vi "Create Queue.vi"() -> ()   [LabVIEW 2015]
uses:
  Core/HTTP Request/Region.ctl
  Core/HTTP Request/AWS Credentials.ctl
  Queue/Queue.lvclass
  Core/HTTP Request/HTTP Request.lvclass
panel:
  in  "Region":T1
  in  "Secret Key":string
  in  "Access Key":string
  in  "Queue Name":string
  # "Overview: Demonstrates how to create a new Amazon SQS queue.\nRequirements: LabVIEW AWS Toolkit and a registered Amazon AWS account\nInstructions:\n1. Specify the Access Key and Secret Key for your AWS account. You can create an account at http://aws.amazon.com.\n2. Specify a Region and Queue Name for the queue you want to create. Note that the queue name must be globally unique.\n3. Run the VI. Verify in the Amazon SQS console that the specified queue was created."
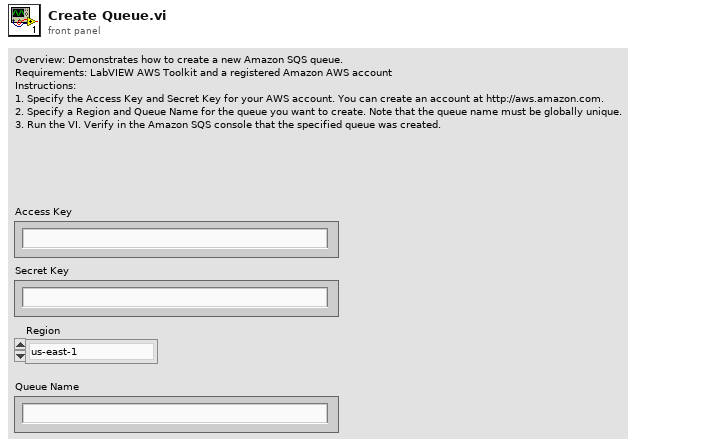
[diagram p1: front panel]
types:
  T1 = typedef "NI_AWS_Core.lvlib/HTTP Request.lvclass/Region.ctl" = enum16{"us-east-1", "us-east-2", "us-west-1", "us-west-2", "ap-northeast-1", "ap-northeast-2", "ap-southeast-1", "ap-southeast-2", "ca-central-1", "eu-central-1", "eu-west-1", "eu-west-2", "sa-east-1"}
  T2 = typedef "NI_AWS_Core.lvlib/HTTP Request.lvclass/AWS Credentials.ctl" = cluster{"Access Key":string, "Secret Key":string}
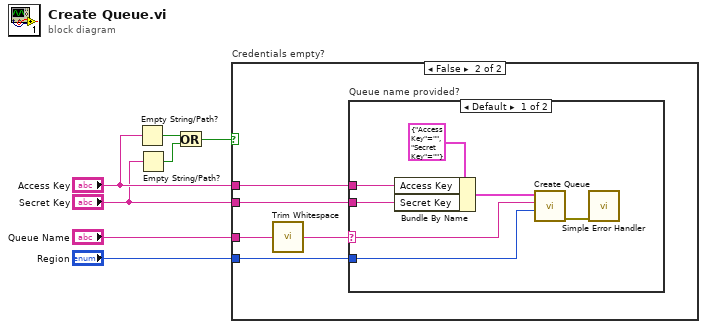
[diagram p0: block diagram]
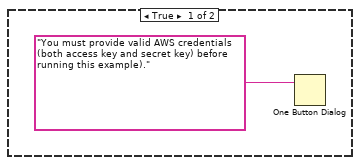
[diagram p2: hidden frame]
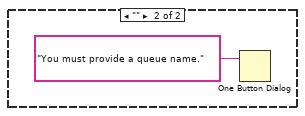
[diagram p3: hidden frame]
diagram:
  n1 = Empty String/Path?(string/path="Access Key") -> (empty?=w7:bool)
  n2 = Empty String/Path?(string/path="Secret Key") -> (empty?=w6:bool)
  n3 = Or(x=w7, y=w6) -> (x .or. y?=w5:bool)
  n4 = case "Credentials empty?" shown="False" w5 {
    tunnel: "Access Key" -> [_ w13]
    tunnel: "Secret Key" -> [_ w12]
    tunnel: "Queue Name" -> [_ w11]
    tunnel: "Region" -> [_ w10]
    frame True {
      n5 = One Button Dialog(message="You must provide valid AWS credentials (both access key and secret key) before running this example).") -> ()  [unwired: 1 in, 1 out]
    }
    frame False {
      n6 = call <vilib>:"Trim Whitespace.vi"("string"=w11) -> ("trimmed string"=w9:string)  [unwired: 1 in]
      n7 = case "Queue name provided?" shown="Default" w9 {
        selector: w9 -> [w15 _]
        tunnel: w13 -> [w18 _]
        tunnel: w12 -> [w17 _]
        tunnel: w10 -> [w16 _]
        frame Default {
          n8 = Bundle By Name(cluster=T2 {"Access Key"="", "Secret Key"=""} ("AWS Credentials"), "Access Key"=w18, "Secret Key"=w17) -> (w20:T2)
          n9 = call "Create Queue.vi"("Region"=w16, "Name"=w15, "AWS Credentials"=w20) -> ("error out"=w14:errorcluster)  [unwired: 7 in, 1 out]
          n10 = call <vilib>:"Simple Error Handler.vi"("error in (no error)"=w14) -> ()  [unwired: 4 in, 5 out]
        }
        frame "" {
          n11 = One Button Dialog(message="You must provide a queue name.") -> ()  [unwired: 1 in, 1 out]
        }
      }
    }
  }
